vi "Read Frame.vi"(8 "error in (no error)":errorcluster, 9 "Read Timeout (ms)":i32=25000, 11 "MJPEG Reader in":refnum<class "MJPEG Reader.lvclass">) -> (0 "error out":errorcluster, 2 "Frame":string, 3 "MJPEG Reader out":refnum<class "MJPEG Reader.lvclass">)   [LabVIEW 2015, in "MJPEG Reader.lvclass"]
uses:
  MJPEG Reader.lvclass
  MJPEG Reader.lvclass/MJPEG Reader.ctl
  Read Frame State.ctl
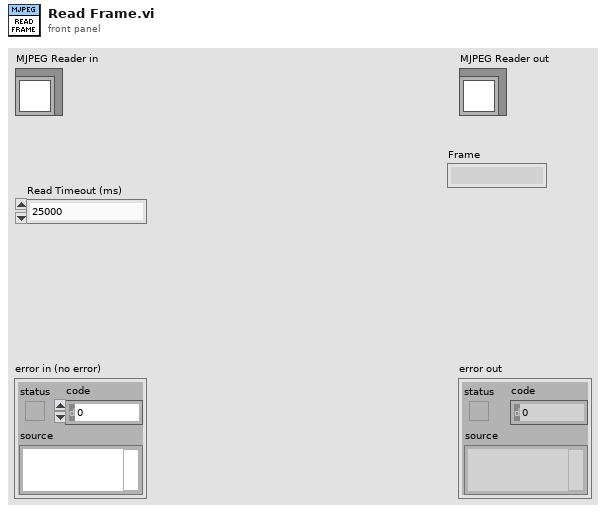
[diagram p1: front panel]
types:
  T1 = typedef "MJPEG Reader.lvclass/Read Frame State.ctl" = enum16{"Wait for Boundary", "Read Headers", "Read Body"}
  T2 = enum16{"Standard", "Buffered", "CRLF", "Immediate"}
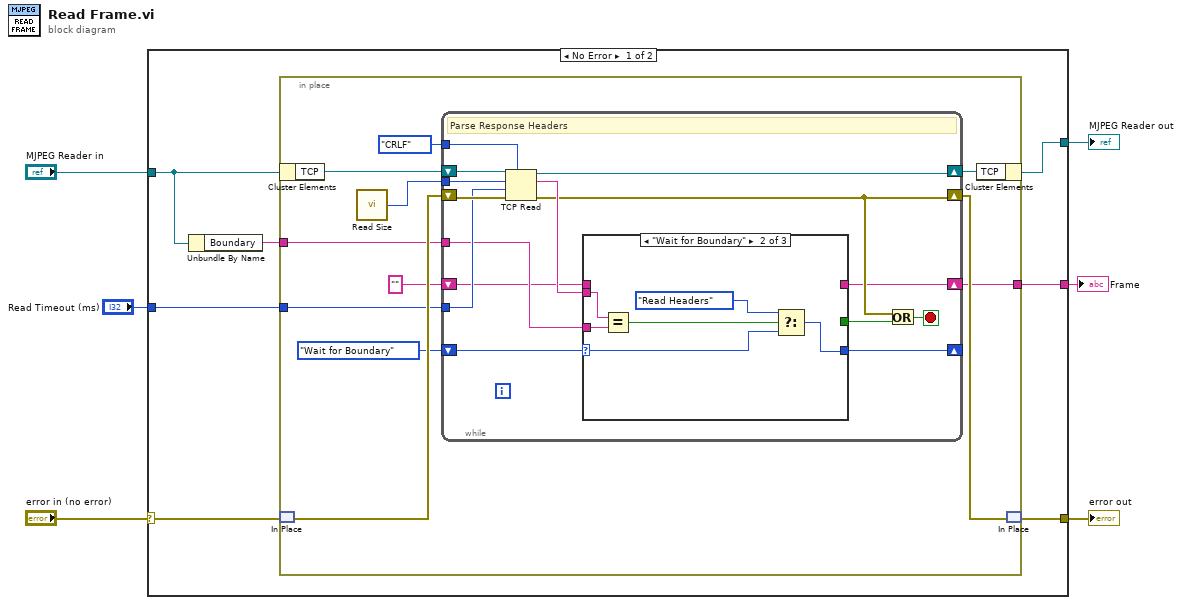
[diagram p0: block diagram]
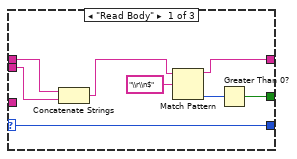
[diagram p2: hidden frame]
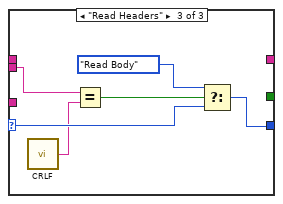
[diagram p3: hidden frame]
diagram:
  n1 = case shown="No Error" "error in (no error)" {
    selector: "error in (no error)" -> [w10 w61]
    tunnel: [w8 w61] -> w5
    tunnel: [w13 w60] -> w3
    tunnel: "MJPEG Reader in" -> [w11 w60]
    tunnel: "Read Timeout (ms)" -> [w12 _]
    tunnel: [w7 _] -> w1
    frame No Error {
      n2 = Unbundle By Name(w11) -> ("Boundary"=w9:string)
      n3 = in-place {
        in-place-border: w12 -> [w19]
        in-place-border: w9 -> [w18]
        in-place-border: [w14] -> w7
        n4 = in-place-cluster #1(w11) -> ("TCP"=w24:refnum<k5>)
        n5 = in-place-match #2(w10) -> (w22:errorcluster)
        n6 = call "Read Size.vi"() -> ("bytes to read"=w20:i32)
        n7 = while {
          shift-right: [w28] -> w17
          shift-left: w22 -> [w38]
          tunnel: T2."CRLF" ("mode (standard)") -> [w37]
          shift-right: [w36] -> w21
          shift-left: w24 -> [w39]
          tunnel: w20 -> [w35]
          tunnel: w19 -> [w34]
          tunnel: w18 -> [w31]
          shift-right: [w30] -> _
          shift-left: Read_Frame_State."Wait for Boundary" ("Read Frame State") -> [w33]
          shift-right: [w25] -> w14
          shift-left: "" -> [w27]
          stop <- w29 stop-if-true
          # "Parse Response Headers"
          n8 = TCP Read(connection ID=w39, bytes to read=w35, error in (no error)=w38, 7:w37, 9:w34) -> (connection ID out=w36:refnum<k5>, data out=w32:string, error out=w28:errorcluster)
          n9 = case shown="\"Wait for Boundary\"" w33 {
            selector: w33 -> [w45 w51 w58]
            tunnel: w32 -> [w46 w53 w59]
            tunnel: w31 -> [_ w52 _]
            tunnel: [w45 w48 w55] -> w30
            tunnel: w27 -> [w47 _ _]
            tunnel: [w44 _ _] -> w26
            tunnel: [w40 _ _] -> w25
            frame "Read Body" {
              n10 = Concatenate Strings(w47, w46) -> (w41:string)
              n11 = Match Pattern(string=w41, regular expression="\\r\\n$") -> (before substring=w40:string, offset past match=w42:i32)  [unwired: 1 in, 2 out]
              n12 = Greater Than 0?(x=w42) -> (x > 0?=w44:bool)
            }
            frame "Wait for Boundary" {
              n13 = Equal?(x=w53, y=w52) -> (x = y?=w50:bool)
              n14 = Select(t=Read_Frame_State."Read Headers", s=w50, f=w51) -> (s? t:f=w48:T1)
            }
            frame "Read Headers" {
              n15 = call "CRLF.vi"() -> ("CRLF"=w54:string)
              n16 = Equal?(x=w59, y=w54) -> (x = y?=w57:bool)
              n17 = Select(t=Read_Frame_State."Read Body", s=w57, f=w58) -> (s? t:f=w55:T1)
            }
          }
          n18 = Or(x=w28, y=w26) -> (x .or. y?=w29:bool)
        }
        n19 = in-place-cluster #1("TCP"=w21) -> (w13:refnum<class "MJPEG Reader.lvclass">)
        n20 = in-place-match #2(w17) -> (w8:errorcluster)
      }
    }
    frame Error {
    }
  }
  "error out" <- w5
  "MJPEG Reader out" <- w3
  "Frame" <- w1
